vi "Get Humidity.vi"(8 "error in (no error)":errorcluster, 10 "Humidity unit":T1(ring), 11 "Sensor General Class in":refnum<class "Sensor General Class.lvclass">) -> (0 "error out":errorcluster, 2 "Temperature":sgl, 3 "Sensor General Class out":refnum<class "Sensor General Class.lvclass">)   [LabVIEW 2020, in "Sensor General Class.lvclass"]
uses:
  Sensor General Class.lvclass
  Data Enum.ctl
  Sensor General Class.lvclass/Sensor General Class.ctl
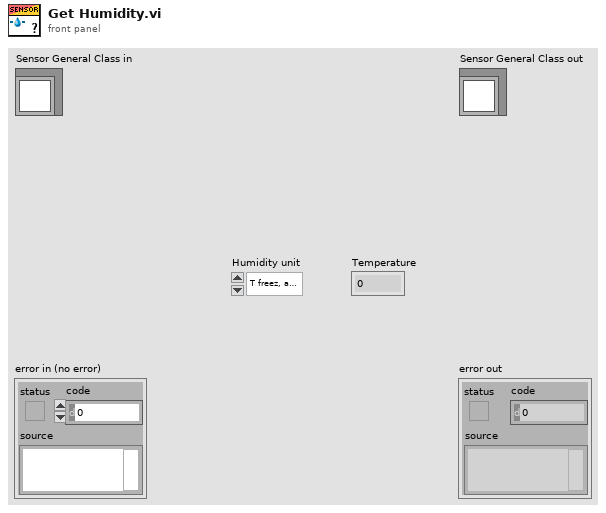
[diagram p1: front panel]
types:
  T1 = enum16{"Т freez, атм, SF6, °C", "Т dew, атм, SF6, °C", "Т freez, бак, SF6, °C", "Т dew, бак, SF6, °C", "Т freez, атм, N2, °C", "Т dew, атм, N2, °C", "Т freez, бак, N2, °C", "Т dew, бак, N2, °C", "ppm(v), SF6", "ppm(w), SF6", "ppm(v), N2", "ppm(w), N2", "rH, %"}
  T2 = typedef "Sensor General Class.lvclass/Data Enum.ctl" = enum16{"p_bar", "p_MPa", "p_Pa", "p_kPa", "p_psi", "p_H/cm^2", "t_C", "t_K", "t_F", "rho_g/l", "rho_kg/m^3", "p20_bar", "related p20_bar", "p20_MPa", "related p20_MPa", "Tf_SF6", "Td_sf6", "tank Tf_SF6", "tank Td_SF6", "Tf_N2", "Td_N2", "tank Tf_N2", "tank Td_N2", "ppm_v SF6", "ppm_w SF6", "ppm_v N2", "ppm_w N2", "rH", "errors"}
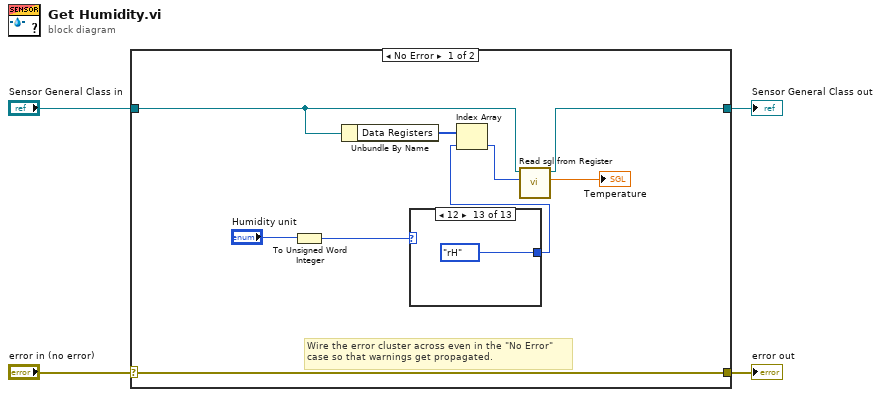
[diagram p0: block diagram]
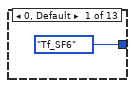
[diagram p2: hidden frame]
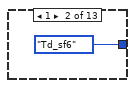
[diagram p3: hidden frame]
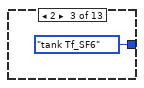
[diagram p4: hidden frame]
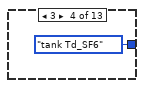
[diagram p5: hidden frame]
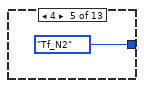
[diagram p6: hidden frame]
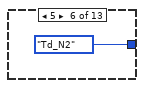
[diagram p7: hidden frame]
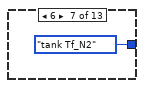
[diagram p8: hidden frame]
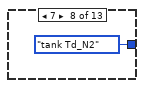
[diagram p9: hidden frame]
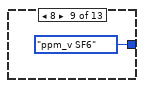
[diagram p10: hidden frame]
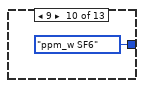
[diagram p11: hidden frame]
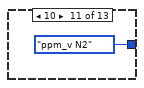
[diagram p12: hidden frame]
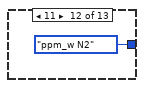
[diagram p13: hidden frame]
diagram:
  n1 = case shown="No Error" "error in (no error)" {
    selector: "error in (no error)" -> [w13 w28]
    tunnel: [w13 w28] -> w3
    tunnel: [w10 w27] -> w1
    tunnel: "Sensor General Class in" -> [w9 w27]
    frame No Error {
      # "Wire the error cluster across even in the \"No Error\"\ncase so that warnings get propagated."
      n2 = To Unsigned Word Integer(number="Humidity unit") -> (unsigned 16bit integer=w6:u16)
      n3 = Unbundle By Name(w9) -> ("Data Registers"=w8:u16[])
      n4 = case shown="12" w6 {
        tunnel: [Data_Enum."Tf_SF6" ("Data Enum") Data_Enum."Td_sf6" ("Data Enum") Data_Enum."tank Tf_SF6" ("Data Enum") Data_Enum."tank Td_SF6" ("Data Enum") Data_Enum."Tf_N2" ("Data Enum") Data_Enum."Td_N2" ("Data Enum") Data_Enum."tank Tf_N2" ("Data Enum") Data_Enum."tank Td_N2" ("Data Enum") Data_Enum."ppm_v SF6" ("Data Enum") Data_Enum."ppm_w SF6" ("Data Enum") Data_Enum."ppm_v N2" ("Data Enum") Data_Enum."ppm_w N2" ("Data Enum") Data_Enum."rH" ("Data Enum")] -> w5
        frame 0, Default {
        }
        frame 1 {
        }
        frame 2 {
        }
        frame 3 {
        }
        frame 4 {
        }
        frame 5 {
        }
        frame 6 {
        }
        frame 7 {
        }
        frame 8 {
        }
        frame 9 {
        }
        frame 10 {
        }
        frame 11 {
        }
        frame 12 {
        }
      }
      n5 = Index Array(array=w8, index=w5) -> (element=w7:u16)
      n6 = call-dynamic "Read sgl from Register.vi"("Start Register"=w7, "Sensor General Class in"=w9) -> ("Data"=→"Temperature":sgl, "Sensor General Class out"=w10:refnum<class "Sensor General Class.lvclass">)  [unwired: 7 in, 1 out]
    }
    frame Error {
    }
  }
  "error out" <- w3
  "Sensor General Class out" <- w1
